vi "RingLocations.vi"(11 "Trans Geometry (mm)":T1={"Transducer"=0, "Geo Focus"=12.0, "a (radius)"=3.0, "# of rings"=5, "kerf space "=0.1, "Center Freq"=12.0} {"Transducer" items=["6D 12R 40 MHz"=0, "10D 31R 20 MHz"=1, "10D 23R 20 MHz"=2, "6D 23R 40 MHz"=3, "4.5D 10.7R 40 MHz"=4, "9D 23.5R 20 MHz"=5, "9D 25.8R 20MHz"=6, "Enter"=99]}) -> (0 "GPU Geometry":dbl[](array[numeric]), 3 "rings (m)":dbl[](array[numeric]))   [LabVIEW 2022 SP3]
uses:
  TransGeometry.ctl
  ArrayGeometry.ctl
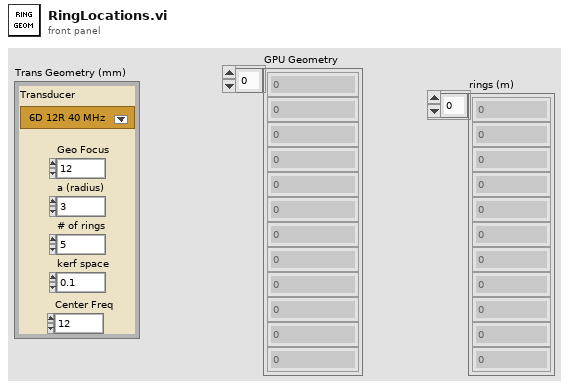
[diagram p1: front panel]
types:
  T1 = typedef "TransGeometry.ctl" = cluster{"Transducer":T2, "Geo Focus":dbl, "a (radius)":dbl, "# of rings":i32, "kerf space ":dbl, "Center Freq":dbl}
  T2 = typedef "ArrayGeometry.ctl" = u16
  T3 = cluster{"Number of rings":i32, "sound spd (cm/s)":i32, "z span (cm)":dbl, "z steps":i32, "y spacing (cm)":dbl, "y steps":i32, "time step (s)":sgl, "z":dbl, "y":dbl, "ref delay":dbl, "freq (MHz)":dbl, "cycles":i32}
  T4 = cluster{"Radius":dbl, "a":dbl, "focus location":dbl}
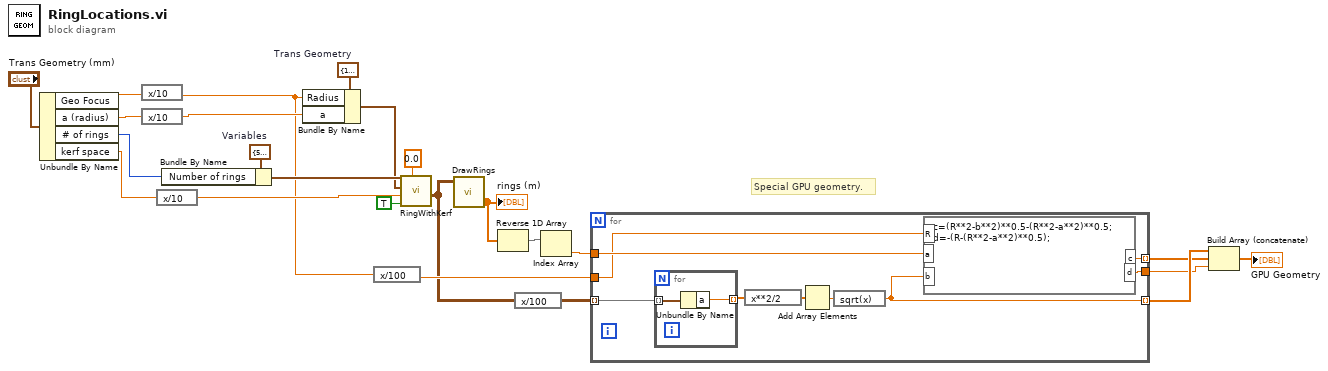
[diagram p0: block diagram]
diagram:
  w21 = T3 {"Number of rings"=5, "sound spd (cm/s)"=150000, "z span (cm)"=4.0, "z steps"=20, "y spacing (cm)"=0.01, "y steps"=50, "time step (s)"=1e-08, "z"=0.0, "y"=0.0, "ref delay"=0.0, "freq (MHz)"=4.71, "cycles"=300}  # Variables
  w19 = T4 {"Radius"=1.2, "a"=0.3, "focus location"=12.0}  # Trans Geometry
  # "Special GPU geometry."
  n1 = Unbundle By Name("Trans Geometry (mm)") -> ("Geo Focus"=w8:dbl, "a (radius)"=w17:dbl, "# of rings"=w20:i32, "kerf space"=w16:dbl)
  n2 = expression code="x/10"(w8) -> (w4:dbl)
  n3 = expression code="x/10"(w17) -> (w18:dbl)
  n4 = expression code="x/10"(w16) -> (w15:dbl)
  n5 = Bundle By Name(cluster=w21, "Number of rings"=w20) -> (w22:T3)
  n6 = Bundle By Name(cluster=w19, "Radius"=w4, "a"=w18) -> (w14:T4)
  n7 = expression code="x/100"(w4) -> (w3:dbl)
  n8 = call "RingWithKerf.vi"("Center Hole"=0.0, "kerf?"=TRUE, "kerf space (cm)"=w15, "Trans Geometry"=w14, "Variables"=w22) -> ("appended array"=w2:cluster{"R":dbl, "a":dbl}[][])  [unwired: 2 in, 2 out]
  n9 = call "DrawRings.vi"("Ring Array"=w2) -> ("rings (m)"=w6:dbl[])  [unwired: 1 in, 7 out]
  "rings (m)" <- w6
  n10 = Reverse 1D Array(array=w6) -> (reversed array=w5:dbl[])
  n11 = expression code="x/100"(w2) -> (w1:cluster{"R":dbl, "a":dbl}[][])
  n12 = Index Array(array=w5) -> (element=w10:dbl)  [unwired: 1 in]
  n13 = for {
    tunnel: [w29] -> w12 mode=indexing
    tunnel: w3 -> [w25]
    tunnel: w10 -> [w32]
    tunnel: [w31] -> w11 mode=indexing
    tunnel: [w28] -> w9
    tunnel: w1 -> [w27] mode=indexing
    n14 = for {
      tunnel: w27 -> [w35] mode=indexing
      tunnel: [w34] -> w26 mode=indexing
      n15 = Unbundle By Name(w35) -> ("a"=w34:dbl)
    }
    n16 = expression code="x**2/2"(w26) -> (w30:dbl[])
    n17 = Add Array Elements(numeric array=w30) -> (sum=w33:dbl)
    n18 = expression code="sqrt(x)"(w33) -> (w29:dbl)
    n19 = formula code="c=(R**2-b**2)**0.5-(R**2-a**2)**0.5;\nd=-(R-(R**2-a**2)**0.5);"("R"=w25, "a"=w32, "b"=w29) -> ("c"=w31:dbl, "d"=w28:dbl)
  }
  n20 = Build Array (concatenate)(w12, w11, w9) -> (→"GPU Geometry":dbl[])
